vi "Continue Processing.vi"(8 "error in (no error)":errorcluster, 10 "Internal Message Queue":refnum<queue>, 11 "TestProcessor in":refnum<class "TestProcessor.lvclass">) -> (0 "error out":errorcluster, 3 "TestProcessor out":refnum<class "TestProcessor.lvclass">)   [LabVIEW 2023, in "HAF.lvlib" / "TestProcessor.lvclass"]
doc: "Ask all Command Directors if they should continue. when all respond false then processing is done. Any that are done will not get processed just because one or more are not yet finished.\n\nAn incoming Stop message that occurs during processing will prevent this state executing as it will be higher in the queue. So a Stop message is only handled once all Command Director Commands have been processed during the current Process state."
uses:
  TestProcessor.lvclass
  Message.ctl
  All Internal Message Ids.ctl
  TestProcessor.lvclass/TestProcessor.ctl
  CommandDirector/CommandDirector.lvclass
  HAF.lvlib
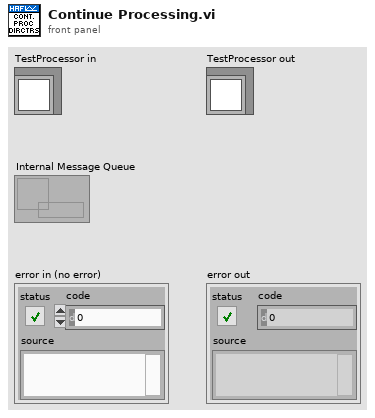
[diagram p1: front panel]
types:
  T1 = typedef "HAF.lvlib/All Internal Message Ids.ctl" = cluster{"Initialise":string, "Process":string, "Continue":string, "Done":string, "Pause":string, "Resume":string, "Stop":string, "Exit":string}
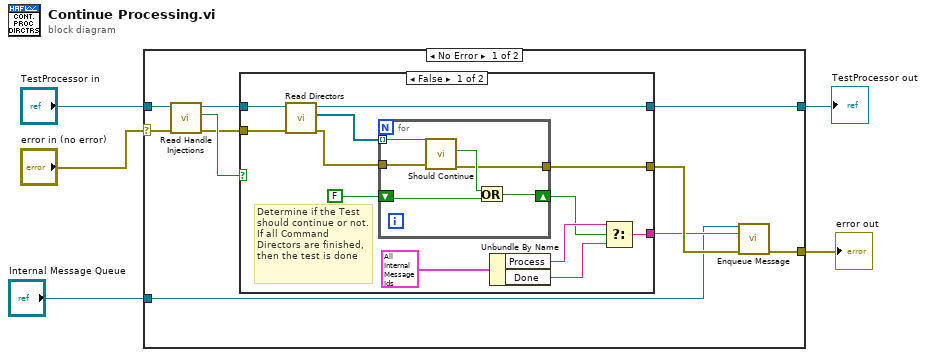
[diagram p0: block diagram]
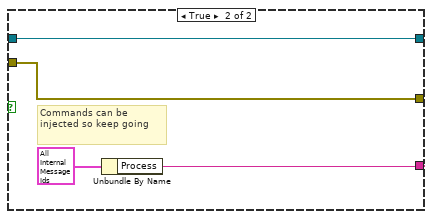
[diagram p2: hidden frame]
diagram:
  n1 = case shown="No Error" "error in (no error)" {
    selector: "error in (no error)" -> [w9 w38]
    tunnel: [w15 w38] -> w5
    tunnel: "Internal Message Queue" -> [w12 _]
    tunnel: [w11 w39] -> w3
    tunnel: "TestProcessor in" -> [w10 w39]
    frame No Error {
      n2 = call-dynamic "Read Handle Injections.vi"("error in (no error)"=w9, "TestProcessor in"=w10) -> ("error out"=w6:errorcluster, "Handle Injections"=w8:bool, "TestProcessor out"=w7:refnum<class "TestProcessor.lvclass">)  [unwired: 7 in]
      n3 = case shown="False" w8 {
        tunnel: [w27 w35] -> w14
        tunnel: [w26 w36] -> w13
        tunnel: [w18 w34] -> w11
        tunnel: w7 -> [w17 w34]
        tunnel: w6 -> [w16 w35]
        frame False {
          # "Determine if the Test should continue or not.  If all Command Directors are finished, then the test is done"
          n4 = call-dynamic "Read Directors.vi"("error in (no error)"=w16, "TestProcessor in"=w17) -> ("error out"=w20:errorcluster, "Directors"=w19:refnum<class "CommandDirector.lvclass">[], "TestProcessor out"=w18:refnum<class "TestProcessor.lvclass">)  [unwired: 7 in]
          n5 = for {
            tunnel: w19 -> [w33] mode=indexing
            tunnel: w20 -> [w32]
            shift-right: [w31] -> w22
            shift-left: FALSE -> [w29]
            tunnel: [w28] -> w27
            n6 = call-dynamic "Should Continue.vi"("error in (no error)"=w32, "CommandDirector in"=w33) -> ("error out"=w28:errorcluster, "Should Continue"=w30:bool)  [unwired: 7 in, 1 out]
            n7 = Or(x=w30, y=w29) -> (x .or. y?=w31:bool)
          }
          n8 = Unbundle By Name(T1 {"Initialise"="Initialise", "Process"="Process", "Continue"="Continue", "Done"="Done", "Pause"="Pause", "Resume"="Resume", "Stop"="Stop", "Exit"="Exit"} ("Message Ids")) -> ("Process"=w24:string, "Done"=w25:string)
          n9 = Select(t=w24, s=w22, f=w25) -> (s? t:f=w26:string)
        }
        frame True {
          # "Commands can be injected so keep going"
          n10 = Unbundle By Name(T1 {"Initialise"="Initialise", "Process"="Process", "Continue"="Continue", "Done"="Done", "Pause"="Pause", "Resume"="Resume", "Stop"="Stop", "Exit"="Exit"} ("Message Ids")) -> ("Process"=w36:string)
        }
      }
      n11 = call "Enqueue Message.vi"("Message Queue In"=w12, "Message Id"=w13, "error in (no error)"=w14) -> ("error out"=w15:errorcluster)  [unwired: 11 in, 1 out]
    }
    frame Error {
    }
  }
  "error out" <- w5
  "TestProcessor out" <- w3
